vi "Delivery Playback.vi"(4 "Home":bool, 5 "Rewind":bool, 7 "Playback":bool, 8 "Taper Limit":dbl=1.0, 9 "Playback allow":bool=TRUE, 10 "Encoder Recording Data":cluster{dbl, u32}[](array[cluster])=[{0.0, 40}, {5.5, 82}, {6.75, 122}, {7.0, 162}, {7.0, 203}, {7.25, 244}, {3.75, 283}, {2.5, 323}, {2.25, 363}, {-0.5, 403}, {-6.75, 444}, {-16.0, 485}, {-28.75, 525}, {-46.0, 565}, {-68.5, 607}, {-94.25, 647}, {-125.25, 689}, {-157.25, 730}, {-189.0, 770}, {-219.75, 811}, {-239.5, 851}, {-265.25, 892}, {-287.0, 932}, {-303.5, 973}, {-312.75, 1014}, {-315.0, 1055}, {-313.5, 1095}, {-306.25, 1136}, {-293.75, 1177}, {-277.0, 1219}, {-254.0, 1261}, {-227.25, 1302}, {-196.0, 1341}, {-158.5, 1382}, {-118.75, 1422}, {-76.75, 1463}, {-36.75, 1503}, {-3.0, 1543}, {26.0, 1583}, {56.5, 1625}, {81.75, 1665}, {100.5, 1706}, {112.5, 1746}, {116.75, 1787}, {116.75, 1828}, {113.0, 1868}, {105.0, 1909}, {92.75, 1949}, {76.25, 1990}, {55.25, 2030}, {29.5, 2071}, {-0.25, 2112}, {-35.25, 2152}, {-74.0, 2193}, {-116.25, 2233}, {-159.0, 2274}, {-202.75, 2314}, {-245.0, 2356}, {-274.5, 2396}, {-310.5, 2436}, {-341.5, 2477}, {-366.25, 2517}, {-383.0, 2558}, {-390.25, 2599}, {-390.75, 2640}, {-387.0, 2681}, {-378.0, 2722}, {-363.0, 2763}, {-343.5, 2804}, {-318.25, 2845}, {-287.0, 2885}, {-248.75, 2926}, {-205.0, 2967}, {-155.75, 3008}, {-102.25, 3049}, {-50.5, 3088}, {1.0, 3130}, {41.25, 3171}, {84.0, 3212}, {122.0, 3253}, {153.75, 3294}, {180.5, 3335}, {200.25, 3375}, {213.5, 3416}, {218.25, 3457}, {218.25, 3496}, {213.5, 3536}, {205.0, 3576}, {192.0, 3617}, {175.0, 3658}, {152.25, 3699}, {125.25, 3740}, {93.5, 3781}, {56.0, 3822}, {13.75, 3863}, {-31.25, 3903}, {-80.25, 3944}, {-130.5, 3986}, {-177.75, 4027}, {-214.25, 4068}, {-253.75, 4108}, {-291.5, 4149}, {-326.0, 4190}, {-356.75, 4231}, {-384.75, 4272}, {-409.5, 4313}, {-431.0, 4353}, {-449.5, 4393}, {-466.0, 4433}, {-479.5, 4474}, {-491.0, 4515}, {-500.0, 4556}, {-506.5, 4597}, {-510.75, 4636}, {-513.0, 4678}, {-513.5, 4718}, {-513.5, 4758}, {-513.5, 4800}, {-513.5, 4840}, {-513.5, 4882}, {-513.5, 4923}, {-513.5, 4964}, {-513.5, 5005}, {-513.5, 5045}, {-513.5, 5085}, {-513.5, 5127}, {-513.5, 5168}, {-513.5, 5211}, {-513.5, 5250}, {-513.5, 5291}, {-513.5, 5331}, {-513.5, 5372}, {-513.5, 5413}, {-513.5, 5454}], 11 "Hardware In":T5={"Motor Selection"="Test motor thing", "EncoderDevRef"={"DevStatus"={"status"=FALSE, "code"=0, "source"=""}, "EncoderIndex"=enum."Enc 0", "CounterIndex"=enum."Invalid", "DistancePerCount"=1.0, "Decoding Type"=enum."4x"}}) -> (0 "Encoder Distance PB":dbl, 1 "Finish Playback":bool)   [LabVIEW 2017]
uses:
  <vilib>/Rock Robotics/WPI/Encoder/WPI_EncoderDevRef.ctl
  <vilib>/Rock Robotics/SystemInterfaces/Encoder/FPGA_EncoderIdx.ctl
  <vilib>/Rock Robotics/SystemInterfaces/Counter/FPGA_CounterCtrSystemIndex.ctl
  <vilib>/Rock Robotics/WPI/Encoder/WPI_EncoderType.ctl
  <vilib>/Rock Robotics/WPI/Utilities/WPI_GetSetVariantRefNum.vi
  <vilib>/addons/control/pid/pid.llb/PID (DBL).vi
  <vilib>/Rock Robotics/WPI/RobotDrive/WPI_RobotDriveArcadeDrive_Standard(NoSaturation).vi
  <vilib>/addons/control/pid/NI_PID_pid.lvlib
panel:
  out "Initial Encoder Position":dbl
  out "Waveform Chart":cluster{dbl, dbl}(graph)
  in  "Playback PID gains":T6={"proportional gain (Kc)"=-0.15, "integral time (Ti, min)"=0.014, "derivative time (Td, min)"=0.0} {"derivative time (Td, min)" format="%.8f"; "integral time (Ti, min)" format="%.8f"; "proportional gain (Kc)" format="%.8f"}
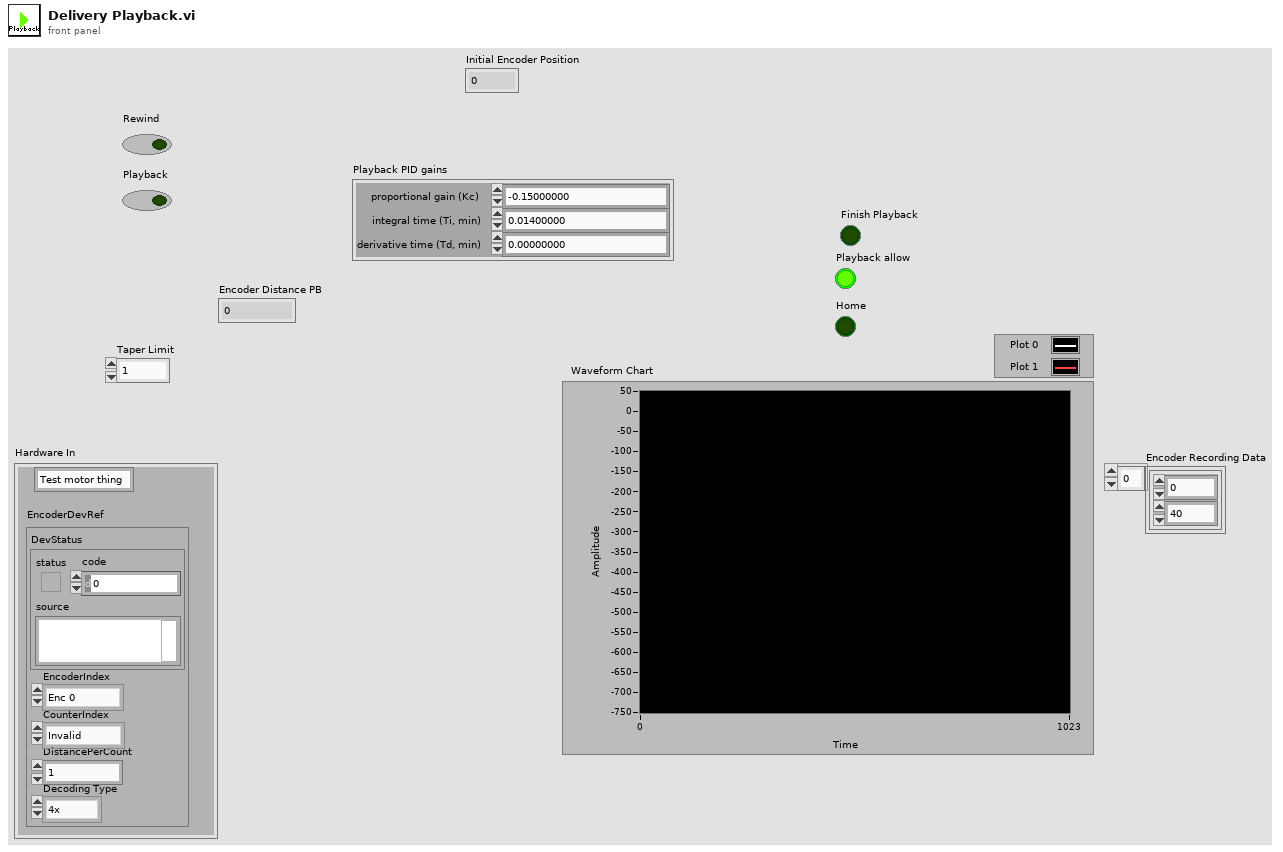
[diagram p1: front panel]
types:
  T1 = typedef "WPI_EncoderDevRef.ctl" = cluster{"DevStatus":errorcluster, "EncoderIndex":T2, "CounterIndex":T3, "DistancePerCount":dbl, "Decoding Type":T4}
  T2 = typedef "FPGA_EncoderIdx.ctl" = enum8{"Enc 0", "Enc 1", "Enc 2", "Enc 3", "Enc 4", "Enc 5", "Enc 6", "Enc 7", "Invalid"}
  T3 = typedef "FPGA_CounterCtrSystemIndex.ctl" = enum8{"Ctr 0", "Ctr 1", "Ctr 2", "Ctr 3", "Ctr 4", "Ctr 5", "Ctr 6", "Ctr 7", "Invalid"}
  T4 = typedef "WPI_EncoderType.ctl" = enum16{"1x", "2x", "4x"}
  T5 = cluster{"Motor Selection":string, "EncoderDevRef":T1}
  T6 = cluster{"proportional gain (Kc)":dbl, "integral time (Ti, min)":dbl, "derivative time (Td, min)":dbl}
  T7 = typedef "WPI_RobotDriveDevRef.ctl" = cluster{"DevStatus":errorcluster, "Motors[]":T8[], "Square Inputs":bool, "Max Output":dbl}
  T8 = typedef "WPI_MotorControlDeviceRef.ctl" = cluster{"DeviceStatus":errorcluster, "Type":T9, "PWM":cluster{"PWM Channel":T10, "DeadBand":T11}, "CAN":cluster{"Device Number":u8, "SetOutput VI Ref":variant, "GetOutput VI Ref":variant, "Enable VI Ref":variant, "Disable VI Ref":variant, "Data":variant}, "Invert":bool, "DIO PWM":cluster{"PWM \"Enable\" Channel":T10, "DIOChannel":T12, "PWM Rate":dbl}}
  T9 = typedef "WPI_MotorControlType.ctl" = enum16{"PWM", "CAN", "DIO PWM"}
  T10 = typedef "FPGA_DIOPWMChannel.ctl" = enum8{"PWM 0", "PWM 1", "PWM 2", "PWM 3", "PWM 4", "PWM 5", "PWM 6", "PWM 7", "PWM 8", "PWM 9", "PWM MXP 0", "PWM MXP 1", "PWM MXP 2", "PWM MXP 3", "PWM MXP 4", "PWM MXP 5", "PWM MXP 6", "PWM MXP 7", "PWM MXP 8", "PWM MXP 9", "Invalid"}
  T11 = typedef "WPI_PWMDeadband.ctl" = cluster{"Name":string, "maxPositivePwm":i32, "minPositivePwm":i32, "centerPwm":i32, "maxNegativePwm":i32, "minNegativePwm":i32, "angularRange":u16}
  T12 = typedef "FPGA_DIOChannel.ctl" = enum8{"DIO 0", "DIO 1", "DIO 2", "DIO 3", "DIO 4", "DIO 5", "DIO 6", "DIO 7", "DIO 8", "DIO 9", "DIO MXP 0", "DIO MXP 1", "DIO MXP 2", "DIO MXP 3", "DIO MXP 4", "DIO MXP 5", "DIO MXP 6", "DIO MXP 7", "DIO MXP 8", "DIO MXP 9", "DIO MXP 10", "DIO MXP 11", "DIO MXP 12", "DIO MXP 13", "DIO MXP 14", "DIO MXP 15", "SPI Port CS1", "SPI Port CS2", "SPI Port CS3", "SPI Port MISO", "SPI Port MOSI", "Invalid"}
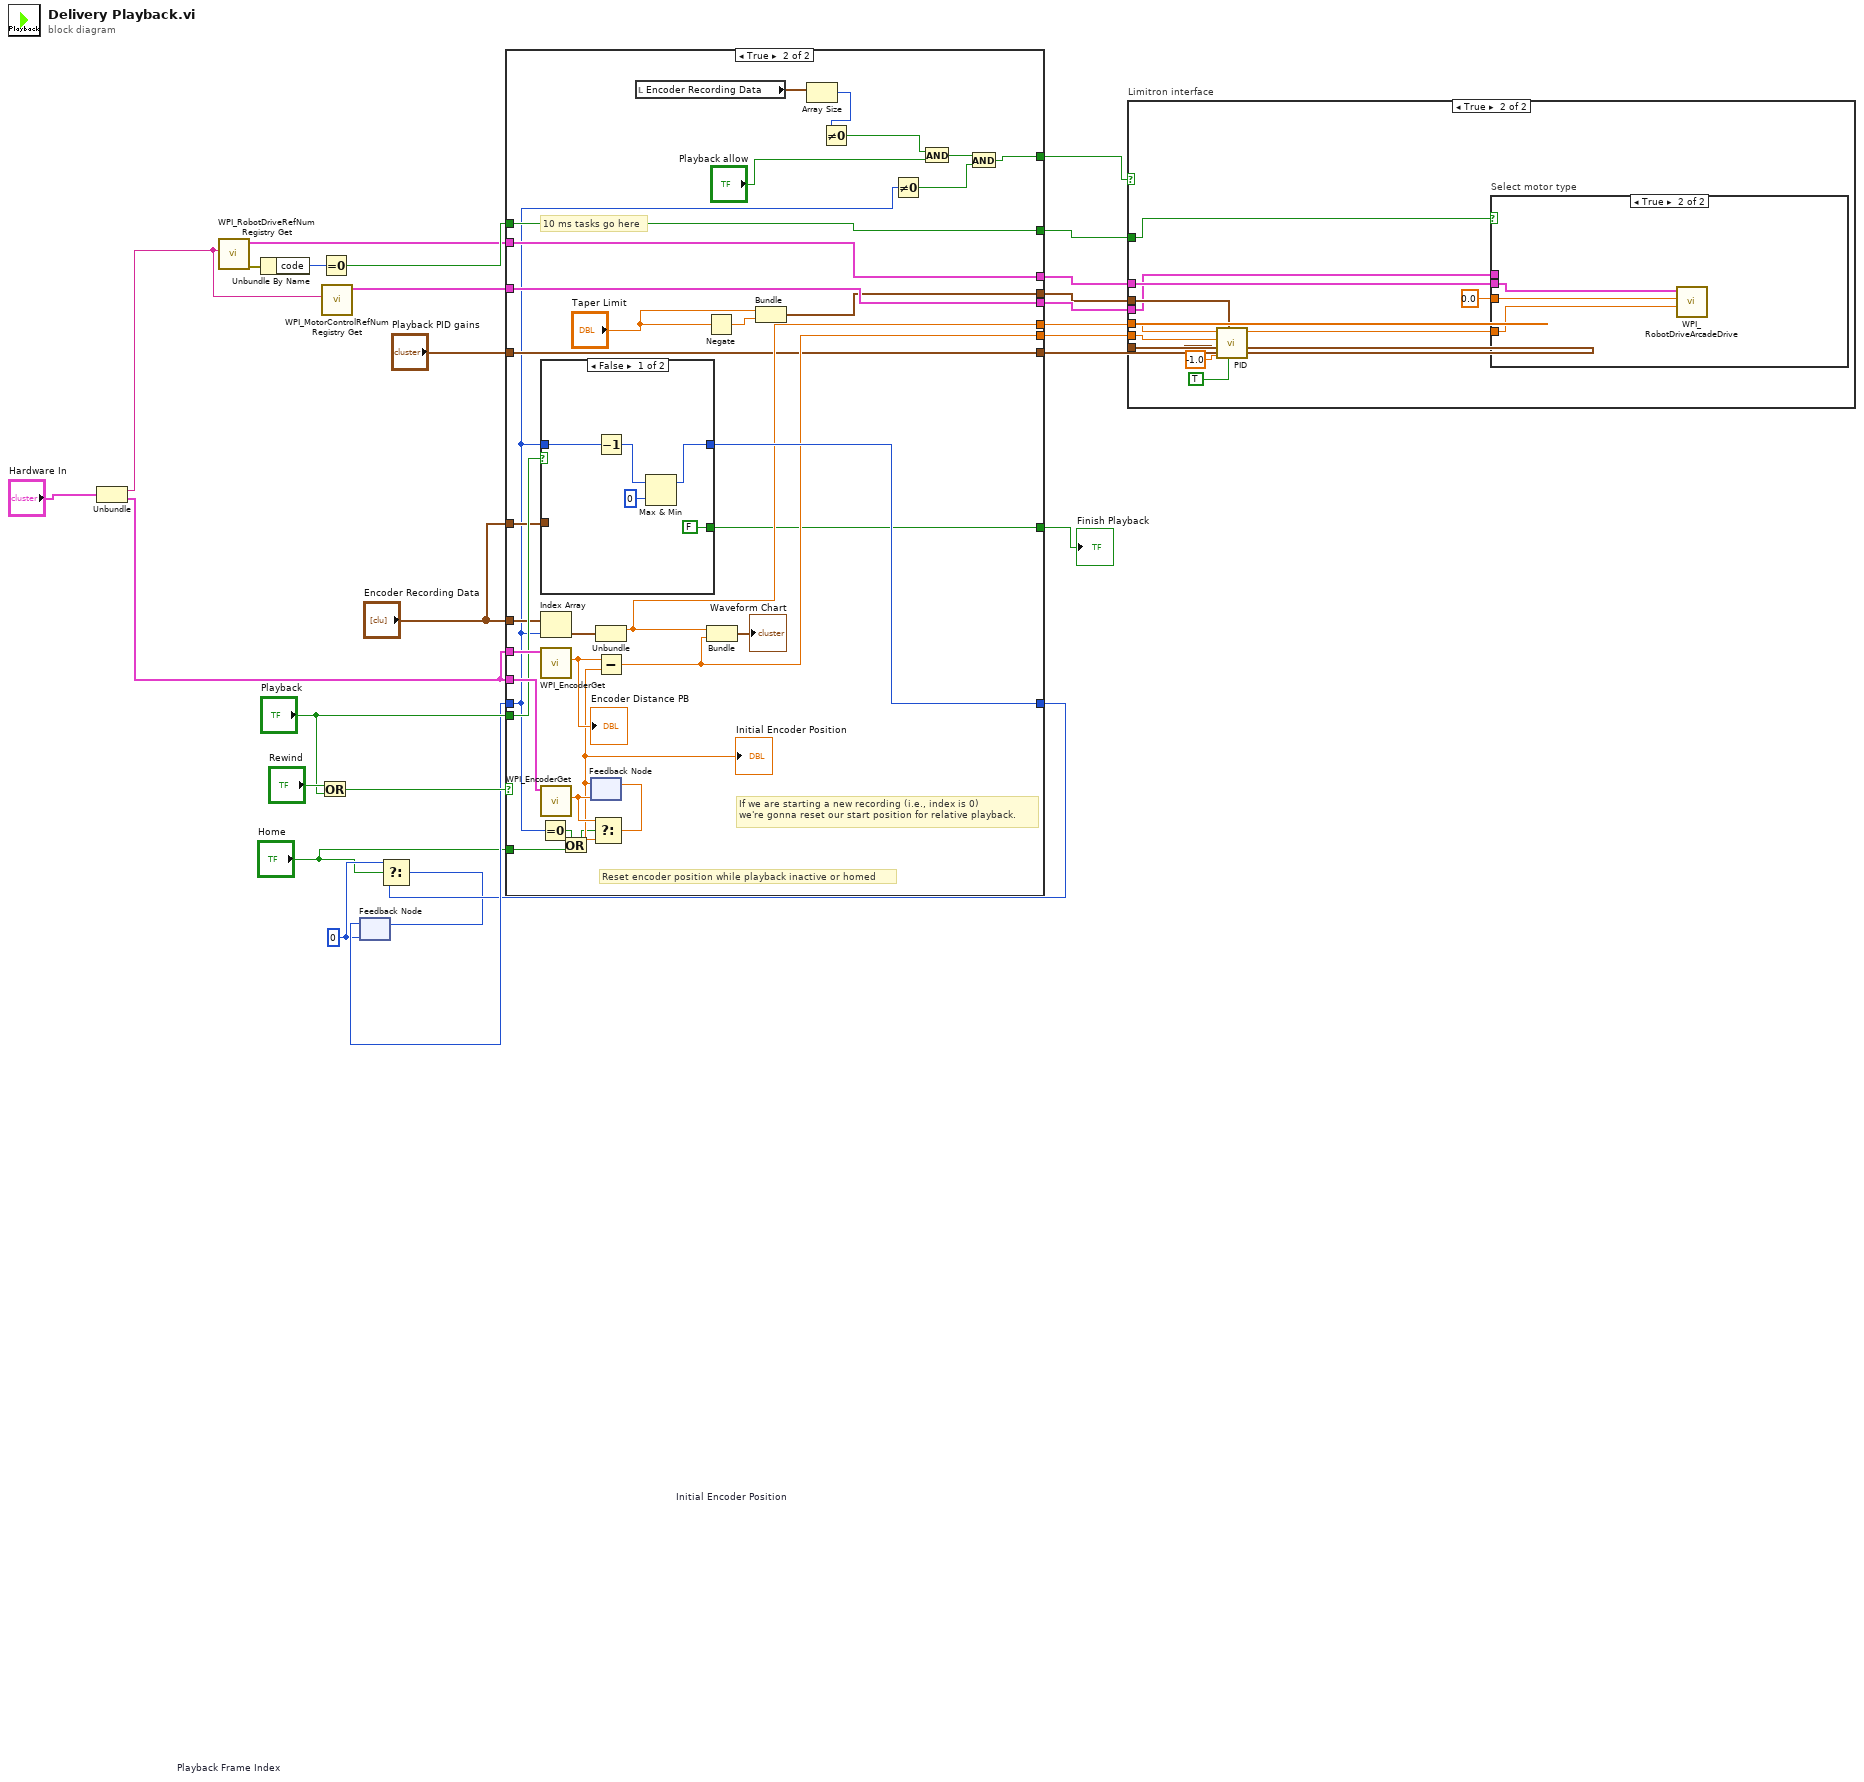
[diagram p0: block diagram]
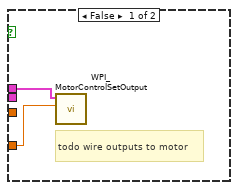
[diagram p3: hidden frame]
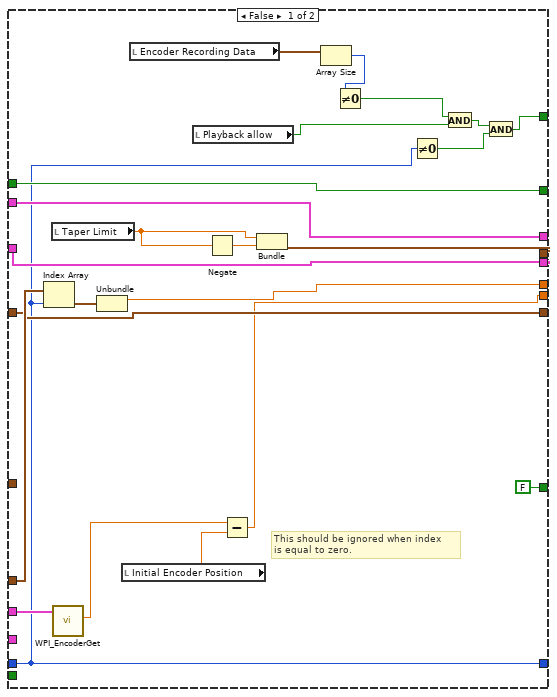
[diagram p4: hidden frame]
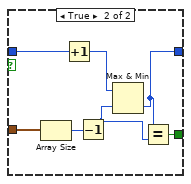
[diagram p5: hidden frame]
diagram:
  w16 = 0 ("index")
  n1 = Unbundle("Hardware In") -> ("Motor Selection"=w12:string, "EncoderDevRef"=w11:T1)
  n2 = call <vilib>:"WPI_RobotDriveRefNum Registry Get.vi"("refnum name"=w12) -> ("error out"=w26:errorcluster, "RobotDriveDevRef"=w24:T7)  [unwired: 1 in, 8 out]
  n3 = Unbundle By Name(w26) -> ("code"=w27:i32)
  n4 = Or(x="Rewind", y="Playback") -> (x .or. y?=w22:bool)
  n5 = Equal To 0?(x=w27) -> (x = 0?=w25:bool)
  n6 = call <vilib>:"WPI_MotorControlRefNum Registry Get.vi"("refnum name"=w12) -> ("MotorControlDevRef"=w20:T8)  [unwired: 9 in, 1 out]
  n7 = feedback #1 "Playback Frame Index"(w16) -> (w19:i32)
  n8 = case shown="True" w22 {
    tunnel: w11 -> [_ w83]
    tunnel: w11 -> [w36 w82]
    tunnel: w25 -> [w46 w70]
    tunnel: w24 -> [w45 w69]
    tunnel: "Playback" -> [_ w81]
    tunnel: w20 -> [w44 w68]
    tunnel: "Encoder Recording Data" -> [w50 w75]
    tunnel: w19 -> [w29 w55]
    tunnel: [w29 w74] -> w17
    tunnel: "Playback PID gains" -> [w42 w64]
    tunnel: "Encoder Recording Data" -> [_ w71]
    tunnel: [w46 w70] -> w10
    tunnel: [w45 w69] -> w9
    tunnel: [w44 w68] -> w8
    tunnel: [w43 w67] -> w7
    tunnel: [w33 w66] -> w6
    tunnel: [w41 w65] -> w5
    tunnel: [w42 w64] -> w4
    tunnel: [w31 w57] -> w3
    tunnel: "Home" -> [_ w52]
    tunnel: [FALSE w51] -> w1
    frame False {
      # "This should be ignored when index \nis equal to zero."
      n9 = Index Array(array=w50, index=w29) -> (element=w49:cluster{dbl, u32})
      n10 = local read "Taper Limit"() -> (w47:dbl)
      n11 = call <vilib>:"WPI_EncoderGet.vi"("EncoderDevRef"=w36) -> ("Distance"=w35:dbl)  [unwired: 5 in, 5 out]
      n12 = Unbundle(w49) -> (w43:dbl)  [unwired: 1 out]
      n13 = local read "Initial Encoder Position"() -> (w34:dbl)
      n14 = local read "Encoder Recording Data"() -> (w37:cluster{dbl, u32}[])
      n15 = local read "Playback allow"() -> (w38:bool)
      n16 = Negate(x=w47) -> (-x=w48:dbl)
      n17 = Subtract(x=w35, y=w34) -> (x-y=w33:dbl)
      n18 = Bundle("Taper Limit"=w47, w48) -> (w41:cluster{"Taper Limit":dbl, dbl})  [unwired: 1 in]
      n19 = Array Size(array=w37) -> (size(s)=w40:i32)
      n20 = Not Equal To 0?(x=w40) -> (x != 0?=w39:bool)
      n21 = Not Equal To 0?(x=w29) -> (x != 0?=w30:bool)
      n22 = And(x=w39, y=w38) -> (x .and. y?=w32:bool)
      n23 = And(x=w32, y=w30) -> (x .and. y?=w31:bool)
    }
    frame True {
      # "Reset encoder position while playback inactive or homed"
      # "If we are starting a new recording (i.e., index is 0)\nwe're gonna reset our start position for relative playback."
      # "10 ms tasks go here"
      n24 = Equal To 0?(x=w55) -> (x = 0?=w54:bool)
      n25 = case shown="False" w81 {
        tunnel: [w85 w90] -> w74
        tunnel: w55 -> [w88 w95]
        tunnel: w71 -> [_ w93]
        tunnel: [FALSE w89] -> w51
        frame False {
          n26 = Decrement(x=w88) -> (x-1=w86:i32)
          n27 = Max & Min(x=w86, y=0) -> (max(x,y)=w85:i32)  [unwired: 1 out]
        }
        frame True {
          n28 = Array Size(array=w93) -> (size(s)=w92:i32)
          n29 = Increment(x=w95) -> (x+1=w94:i32)
          n30 = Decrement(x=w92) -> (x-1=w91:i32)
          n31 = Max & Min(x=w94, y=w91) -> (min(x,y)=w90:i32)  [unwired: 1 out]
          n32 = Equal?(x=w90, y=w91) -> (x = y?=w89:bool)
        }
      }
      n33 = Index Array(array=w75, index=w55) -> (element=w76:cluster{dbl, u32})
      n34 = call <vilib>:"WPI_EncoderGet.vi"("EncoderDevRef"=w82) -> ("Distance"=w80:dbl)  [unwired: 5 in, 5 out]
      "Encoder Distance PB" <- w80
      n35 = call <vilib>:"WPI_EncoderGet.vi"("EncoderDevRef"=w83) -> ("Distance"=w73:dbl)  [unwired: 5 in, 5 out]
      n36 = Or(x=w54, y=w52) -> (x .or. y?=w53:bool)
      n37 = feedback #2 "Initial Encoder Position"(w73) -> (w72:dbl)
      "Initial Encoder Position" <- w72
      n38 = Select(t=w73, s=w53, f=w72) -> (s? t:f=w59:dbl)
      n39 = feedback-in #2(w59) -> ()
      n40 = Unbundle(w76) -> (w67:dbl)  [unwired: 1 out]
      n41 = Subtract(x=w80, y=w72) -> (x-y=w66:dbl)
      n42 = local read "Encoder Recording Data"() -> (w62:cluster{dbl, u32}[])
      n43 = Negate(x="Taper Limit") -> (-x=w78:dbl)
      n44 = Bundle(w67, w66) -> (→"Waveform Chart":cluster{dbl, dbl})  [unwired: 1 in]
      n45 = Bundle("Taper Limit"="Taper Limit", w78) -> (w65:cluster{"Taper Limit":dbl, dbl})  [unwired: 1 in]
      n46 = Array Size(array=w62) -> (size(s)=w63:i32)
      n47 = Not Equal To 0?(x=w63) -> (x != 0?=w60:bool)
      n48 = Not Equal To 0?(x=w55) -> (x != 0?=w56:bool)
      n49 = And(x=w60, y="Playback allow") -> (x .and. y?=w58:bool)
      n50 = And(x=w58, y=w56) -> (x .and. y?=w57:bool)
    }
  }
  "Finish Playback" <- w1
  n51 = Select(t=w16, s="Home", f=w17) -> (s? t:f=w15:i32)
  n52 = feedback-in #1(w15) -> ()
  n53 = case "Limitron interface" shown="True" w3 {
    tunnel: w4 -> [_ w106]
    tunnel: w6 -> [_ w103]
    tunnel: w7 -> [_ w102]
    tunnel: w8 -> [_ w97]
    tunnel: w10 -> [_ w98]
    tunnel: w9 -> [_ w100]
    tunnel: w5 -> [_ w99]
    frame False {
    }
    frame True {
      n54 = call-poly <vilib>:"PID.vi"("reinitialize? (F)"=TRUE, "output range"=w99, "dt (s)"=-1.0, "PID gains"=w106, "process variable"=w103, "setpoint"=w102) -> ("output"=w101:dbl)  [unwired: 4 in, 1 out]
      n55 = case "Select motor type" shown="True" w98 {
        tunnel: 0.0 ("output") -> [_ w111]
        tunnel: w101 -> [w108 w110]
        tunnel: w100 -> [_ w109]
        tunnel: w97 -> [w107 _]
        frame False {
          # "todo wire outputs to motor"
          n56 = call <vilib>:"WPI_MotorControlSetOutput.vi"("Output"=w108, "MotorControlDevRef"=w107) -> ()  [unwired: 7 in, 3 out]
        }
        frame True {
          n57 = call-poly <vilib>:"WPI_RobotDriveArcadeDrive.vi"("Y axis value"=w110, "X axis value"=w111, "RobotDriveDevRef"=w109) -> ()  [unwired: 6 in, 3 out]
        }
      }
    }
  }
